vi "Macro.vi"(2 "Tasks in":T2={"inbits"=8, "outbits"=38, "Counter"="Counter", "Inbits"="Inbits", "Outbits"="Outbits", "Fast AO"=["FastAO_1", "FastAO_2"], "Errors"={"status"=FALSE, "code"=0, "source"=""}}, 3 "Macro Instructions":T1, 4 "PhiCorrect_RAW":i16=773) -> (1 "Tasks out":T2={"inbits"=8, "outbits"=38, "Counter"="Counter", "Inbits"="Inbits", "Outbits"="Outbits", "Fast AO"=["FastAO_1", "FastAO_2"], "Errors"={"status"=FALSE, "code"=0, "source"=""}})   [LabVIEW 2018]
uses:
  Target/Tasks_RT.ctl
  Instructions_RT.ctl
  <vilib>/DAQmx/write.llb/DAQmx Write (Raw 1D I16).vi
  <vilib>/DAQmx/write.llb/DAQmx Write (Digital 1D Bool 1Chan 1Samp).vi
  <vilib>/DAQmx/miscellaneous.llb/DAQmx Fill In Error Info.vi
  <resource>/objmgr/daqmx.rc
panel:
  # "Tasks and errors"
  # "Tasks and errors"
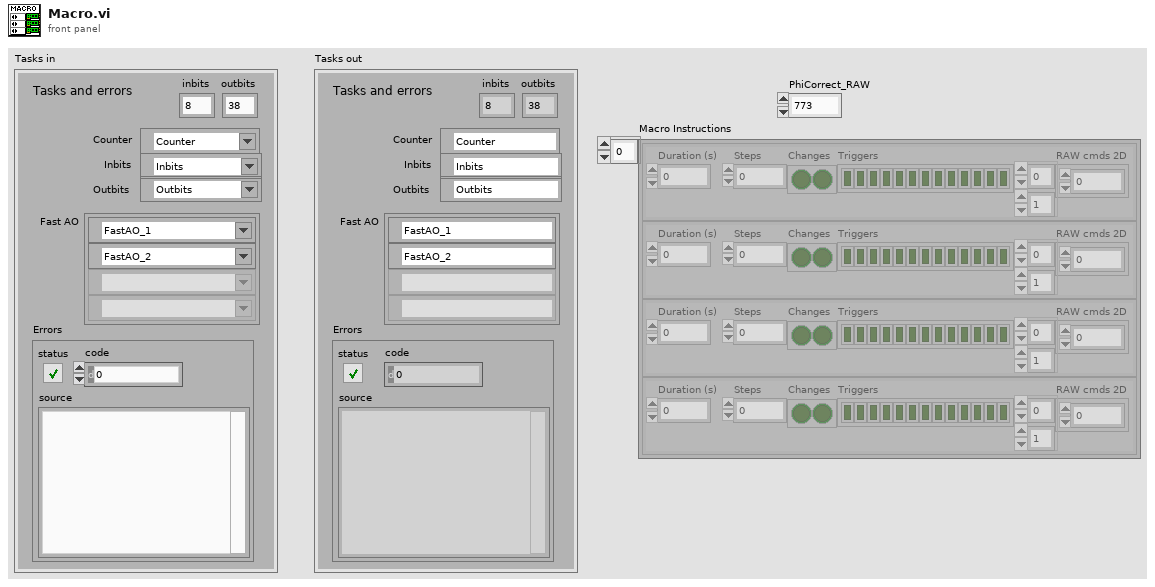
[diagram p1: front panel]
types:
  T1 = typedef "Instructions_RT.ctl" = cluster{"Duration (s)":dbl, "Steps":i32, "Changes":bool[], "Triggers":bool[], "RAW cmds 2D":i16[][]}[]
  T2 = typedef "Tasks_RT.ctl" = cluster{"inbits":i32, "outbits":i32, "Counter":refnum<k21>, "Inbits":refnum<k21>, "Outbits":refnum<k21>, "Fast AO":refnum<k21>[], "Errors":errorcluster}
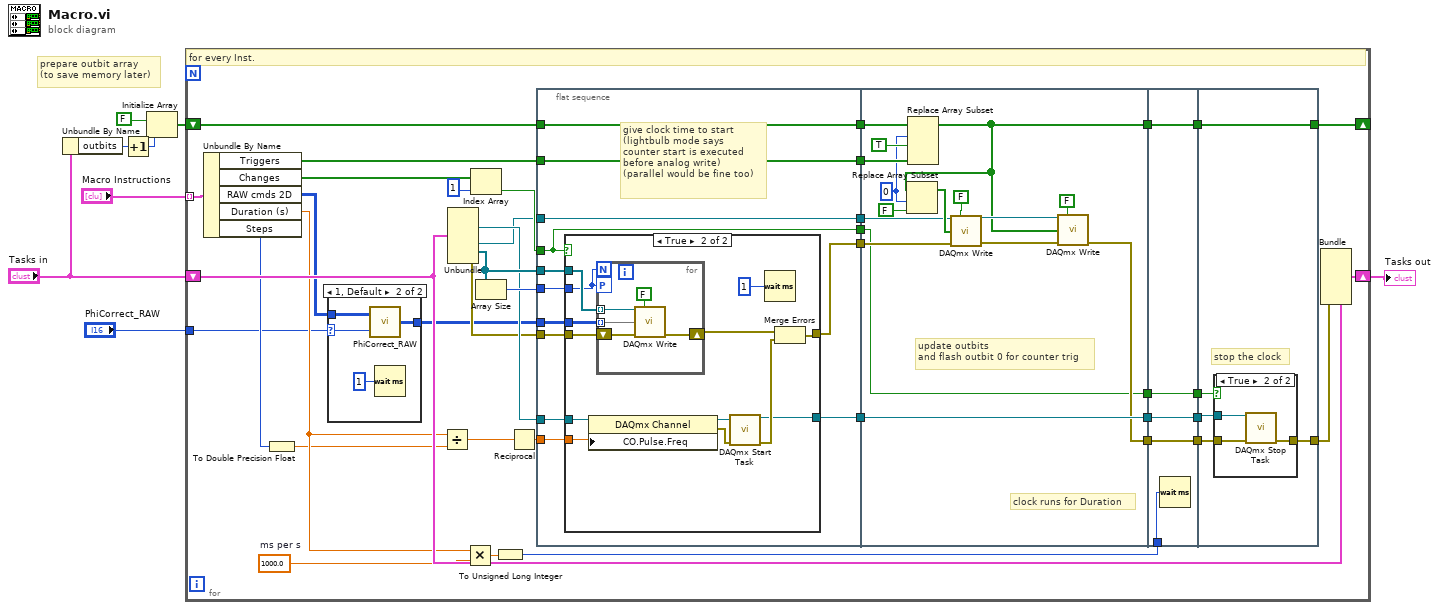
[diagram p0: block diagram]
diagram:
  # "prepare outbit array \n(to save memory later)"
  n1 = Unbundle By Name("Tasks in") -> ("outbits"=w3:i32)
  n2 = Increment(x=w3) -> (x+1=w4:i32)
  n3 = Initialize Array(FALSE ("auto start"), w4) -> (w2:bool[])
  n4 = for {
    tunnel: "Macro Instructions" -> [w48] mode=indexing
    shift-right: [w45] -> w7
    shift-left: "Tasks in" -> [w46]
    shift-right: [w19] -> _
    shift-left: w2 -> [w31]
    tunnel: "PhiCorrect_RAW" -> [w9]
    w40 = 1000.0  # ms per s
    # "for every Inst."
    n5 = Unbundle By Name(w48) -> ("Triggers"=w41:bool[], "Changes"=w42:bool[], "RAW cmds 2D"=w11:i16[][], "Duration (s)"=w39:dbl, "Steps"=w22:i32)
    n6 = To Double Precision Float(number=w22) -> (double precision float=w26:dbl)
    n7 = case shown="1, Default" w9 {
      selector: w9 -> [_ w113]
      tunnel: [w111 w114] -> w10
      tunnel: w11 -> [w111 w115]
      frame 0 {
      }
      frame 1, Default {
        n8 = call "PhiCorrect_RAW.vi"("PhiCorrect_RAW"=w113, "RAW cmds 2D in"=w115) -> ("RAW cmds 2D out"=w114:i16[][])
        n9 = Wait (ms)(milliseconds to wait=u32 1) -> ()  [unwired: 1 out]
      }
    }
    n10 = Divide(x=w39, y=w26) -> (x/y=w18:dbl)
    n11 = Unbundle(w46) -> ("Counter"=w35:refnum<k21>, "Outbits"=w33:refnum<k21>, "Fast AO"=w36:refnum<k21>[], "Errors"=w34:errorcluster)  [unwired: 3 out]
    n12 = Multiply(x=w39, y=w40) -> (x*y=w38:dbl)
    n13 = Index Array(array=w42, index=1) -> (element=w44:bool)
    n14 = Array Size(array=w36) -> (size(s)=w43:i32)
    n15 = To Unsigned Long Integer(number=w38) -> (unsigned 32bit integer=w23:u32)
    n16 = Reciprocal(x=w18) -> (1/x=w37:dbl)
    n17 = flat-sequence {
      tunnel: w44 -> [w49]
      tunnel: w10 -> [w60]
      tunnel: w36 -> [w59]
      tunnel: w34 -> [w58]
      tunnel: w35 -> [w57]
      tunnel: w43 -> [w56]
      tunnel: w37 -> [w55]
      tunnel: w41 -> [w52]
      tunnel: [w52] -> w13
      tunnel: w33 -> [w51]
      tunnel: [w51] -> w14
      tunnel: [w54] -> w15
      tunnel: [w53] -> w16
      tunnel: [w50] -> w17
      tunnel: w31 -> [w50]
      tunnel: [w49] -> w12
      tunnel: [w96] -> w30
      tunnel: [w95] -> w28
      tunnel: w17 -> [w86]
      tunnel: w16 -> [w96]
      tunnel: w15 -> [w88]
      tunnel: w14 -> [w89]
      tunnel: w13 -> [w85]
      tunnel: w12 -> [w82]
      tunnel: [w82] -> w25
      tunnel: [w81] -> w20
      tunnel: w30 -> [w101]
      tunnel: [w101] -> w29
      tunnel: w28 -> [w100]
      tunnel: [w100] -> w27
      tunnel: w23 -> [w99]
      tunnel: w25 -> [w98]
      tunnel: [w98] -> w24
      tunnel: [w97] -> w21
      tunnel: w20 -> [w97]
      tunnel: [w104] -> w32
      tunnel: w29 -> [w106]
      tunnel: w27 -> [w105]
      tunnel: w24 -> [w103]
      tunnel: [w102] -> w19
      tunnel: w21 -> [w102]
      frame #0 {
        # "give clock time to start\n(lightbulb mode says\ncounter start is executed\nbefore analog write)\n(parallel would be fine too)"
        n18 = case shown="True" w49 {
          tunnel: w60 -> [_ w74]
          tunnel: w59 -> [_ w70]
          tunnel: w58 -> [w62 w75]
          tunnel: [w62 w65] -> w54
          tunnel: w57 -> [w61 w71]
          tunnel: [w61 w64] -> w53
          tunnel: w56 -> [_ w69]
          tunnel: w55 -> [_ w68]
          frame False {
          }
          frame True {
            n19 = property class="DAQmx Channel"(reference=w71, "CO.Pulse.Freq"=w68) -> (reference out=w73:refnum<k21>, error out=w72:errorcluster)  [unwired: 1 in]
            n20 = for {
              N: w69 -> [_]
              tunnel: w74 -> [w77] mode=indexing
              tunnel: w70 -> [w78] mode=indexing
              workers-P: w69 -> [_]
              shift-right: [w76] -> w67
              shift-left: w75 -> [w80]
              n21 = call-poly <vilib>:"DAQmx Write.vi"("task/channels in"=w78, "auto start"=FALSE, "data"=w77, "error in"=w80) -> ("error out"=w76:errorcluster)  [unwired: 9 in, 2 out]
            }
            n22 = call <vilib>:"DAQmx Start Task.vi"("task/channels in"=w73, "error in"=w72) -> ("task out"=w64:refnum<k21>, "error out"=w66:errorcluster)  [unwired: 12 in]
            n23 = Wait (ms)(milliseconds to wait=u32 1) -> ()  [unwired: 1 out]
            n24 = Merge Errors(w67, w66) -> (w65:errorcluster)
          }
        }
      }
      frame #1 {
        w83 = 0 ("index")
        # "clock runs for Duration"
        # "update outbits \nand flash outbit 0 for counter trig"
        n25 = Replace Array Subset(array=w86, new element #1=TRUE ("OK Button"), index #1=w83, new element #2=w85) -> (w81:bool[])  [unwired: 1 in]
        n26 = Replace Array Subset(array=w81, new element=FALSE ("OK Button"), index=w83) -> (w93:bool[])
        n27 = call-poly <vilib>:"DAQmx Write.vi"("task/channels in"=w89, "auto start"=FALSE, "data"=w93, "error in"=w88) -> ("task out"=w92:refnum<k21>, "error out"=w91:errorcluster)  [unwired: 9 in, 1 out]
        n28 = call-poly <vilib>:"DAQmx Write.vi"("task/channels in"=w92, "auto start"=FALSE, "data"=w81, "error in"=w91) -> ("error out"=w95:errorcluster)  [unwired: 9 in, 2 out]
      }
      frame #2 {
        n29 = Wait (ms)(milliseconds to wait=w99) -> ()  [unwired: 1 out]
      }
      frame #3 {
        # "stop the clock"
        n30 = case shown="True" w103 {
          tunnel: w106 -> [_ w110]
          tunnel: w105 -> [w107 w109]
          tunnel: [w107 w108] -> w104
          frame False {
          }
          frame True {
            n31 = call <vilib>:"DAQmx Stop Task.vi"("task/channels in"=w110, "error in"=w109) -> ("error out"=w108:errorcluster)  [unwired: 12 in, 1 out]
          }
        }
      }
    }
    n32 = Bundle(cluster=w46, "Errors"=w32) -> (w45:T2)  [unwired: 6 in]
  }
  "Tasks out" <- w7
